vi "读取计数值.vi"(8 "error in (no error)":errorcluster, 10 "通道":T1(ring), 11 "MB session in":refnum<class "MB_Master.lvclass">) -> (0 "error out":errorcluster, 2 "计数值":i32, 3 "MB session out":refnum<class "MB_Master.lvclass">)   [LabVIEW 2016, in "DAM395CF.lvlib"]
uses:
  DAM395CF.lvlib
  <vilib>/Plasmionique/MB Master/MB_Master/MB_Master.lvclass
  <vilib>/Plasmionique/MB Master/MB Master.lvlib
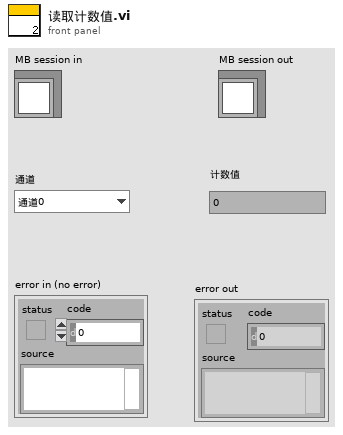
[diagram p1: front panel]
types:
  T1 = enum16{"通道0", "通道1", "通道2", "通道3", "通道4", "通道5", "通道6", "通道7"}
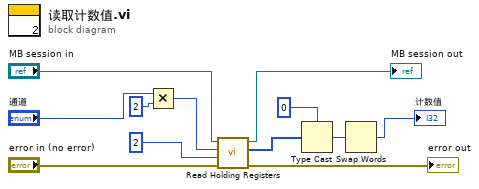
[diagram p0: block diagram]
diagram:
  n1 = Multiply(x="通道", y=2) -> (x*y=w7:i32)
  n2 = call <vilib>:"Read Holding Registers.vi"("error in (no error)"="error in (no error)", "quantity"=u16 2 ("starting address"), "starting address"=w7, "MB session in"="MB session in") -> ("error out"=→"error out":errorcluster, "Registers"=w5:u16[], "MB session out"=→"MB session out":refnum<class "MB_Master.lvclass">)  [unwired: 5 in]
  n3 = Type Cast(type=0, x=w5) -> (*(type *) &x=w3:i32)
  n4 = Swap Words(1:w3) -> (0:→"计数值":i32)
